vi "AprilTagFieldLayout_New2026Welded.vi"() -> (3 "AprilTagFieldLayout":T1={"AprilTagMap"={}, "FieldLength"=0.0, "FieldWidth"=0.0, "OriginPosition "=enum."kBlueAllianceWallRightSide,", "OriginPose3d"={"Translation3d"={"X"=0.0, "Y"=0.0, "Z"=0.0}, "Rotation3d"={"Q_quaternion"={"R"=1.0, "V"=[0.0, 0.0, 0.0]}}}} {"OriginPose3d"."Translation3d"."Z" format="%14.3f"; "OriginPose3d"."Translation3d"."Y" format="%14.3f"; "OriginPose3d"."Translation3d"."X" format="%14.3f"})   [LabVIEW 2019, in "Trajectory_Library.lvlib"]
doc: "Define the FRC 2026 April Tag field layout.\n\nInputs:\n <none>\n\nOutputs:\n -- AprilTagFieldLayout -- AprilTagFieldLayout -- Data cluster containing field definition."
uses:
  TypeDef/AprilTagFieldLayout.ctl
  TypeDef/AprilTag.ctl
  TypeDef/POSE3D.ctl
  TypeDef/TRANSLATION3D.ctl
  TypeDef/ROTATION3D.ctl
  TypeDef/QUATERNION.ctl
  Enum/AprilTagFieldLayoutOrignPosition_ENUM.ctl
  AprilTag_GetAll.vi
  Quaternion_Normalize.vi
  Quaternion_New_Default.vi
  Trajectory_Library.lvlib
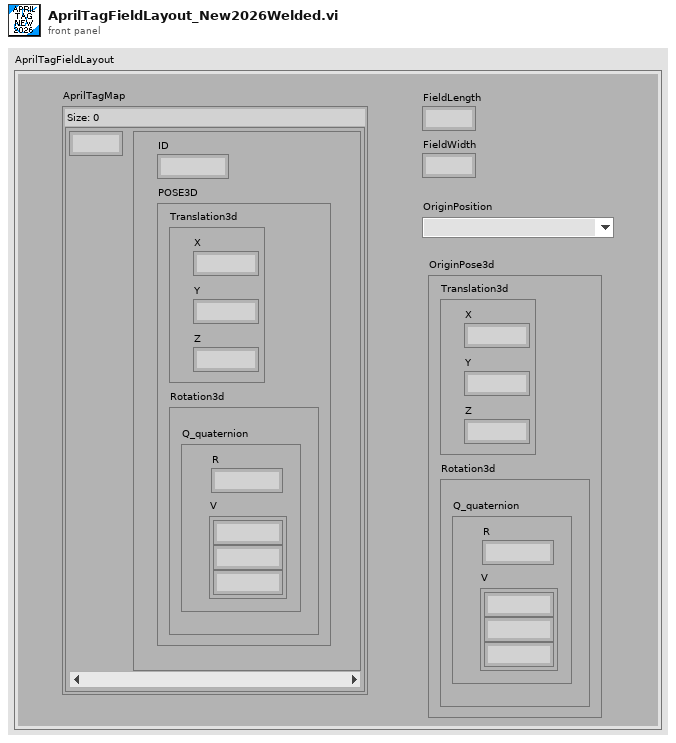
[diagram p1: front panel]
types:
  T1 = typedef "Trajectory_Library.lvlib/AprilTagFieldLayout.ctl" = cluster{"AprilTagMap":map{i32, T2}, "FieldLength":dbl, "FieldWidth":dbl, "OriginPosition ":T7, "OriginPose3d":T3}
  T2 = typedef "Trajectory_Library.lvlib/AprilTag.ctl" = cluster{"ID":i32, "POSE3D":T3}
  T3 = typedef "Trajectory_Library.lvlib/POSE3D.ctl" = cluster{"Translation3d":T4, "Rotation3d":T5}
  T4 = typedef "Trajectory_Library.lvlib/TRANSLATION3D.ctl" = cluster{"X":dbl, "Y":dbl, "Z":dbl}
  T5 = typedef "Trajectory_Library.lvlib/ROTATION3D.ctl" = cluster{"Q_quaternion":T6}
  T6 = typedef "Trajectory_Library.lvlib/QUATERNION.ctl" = cluster{"R":dbl, "V":dbl[]}
  T7 = typedef "Trajectory_Library.lvlib/AprilTagFieldLayoutOrignPosition_ENUM.ctl" = enum16{"kBlueAllianceWallRightSide,", "kRedAllianceWallRightSide,"}
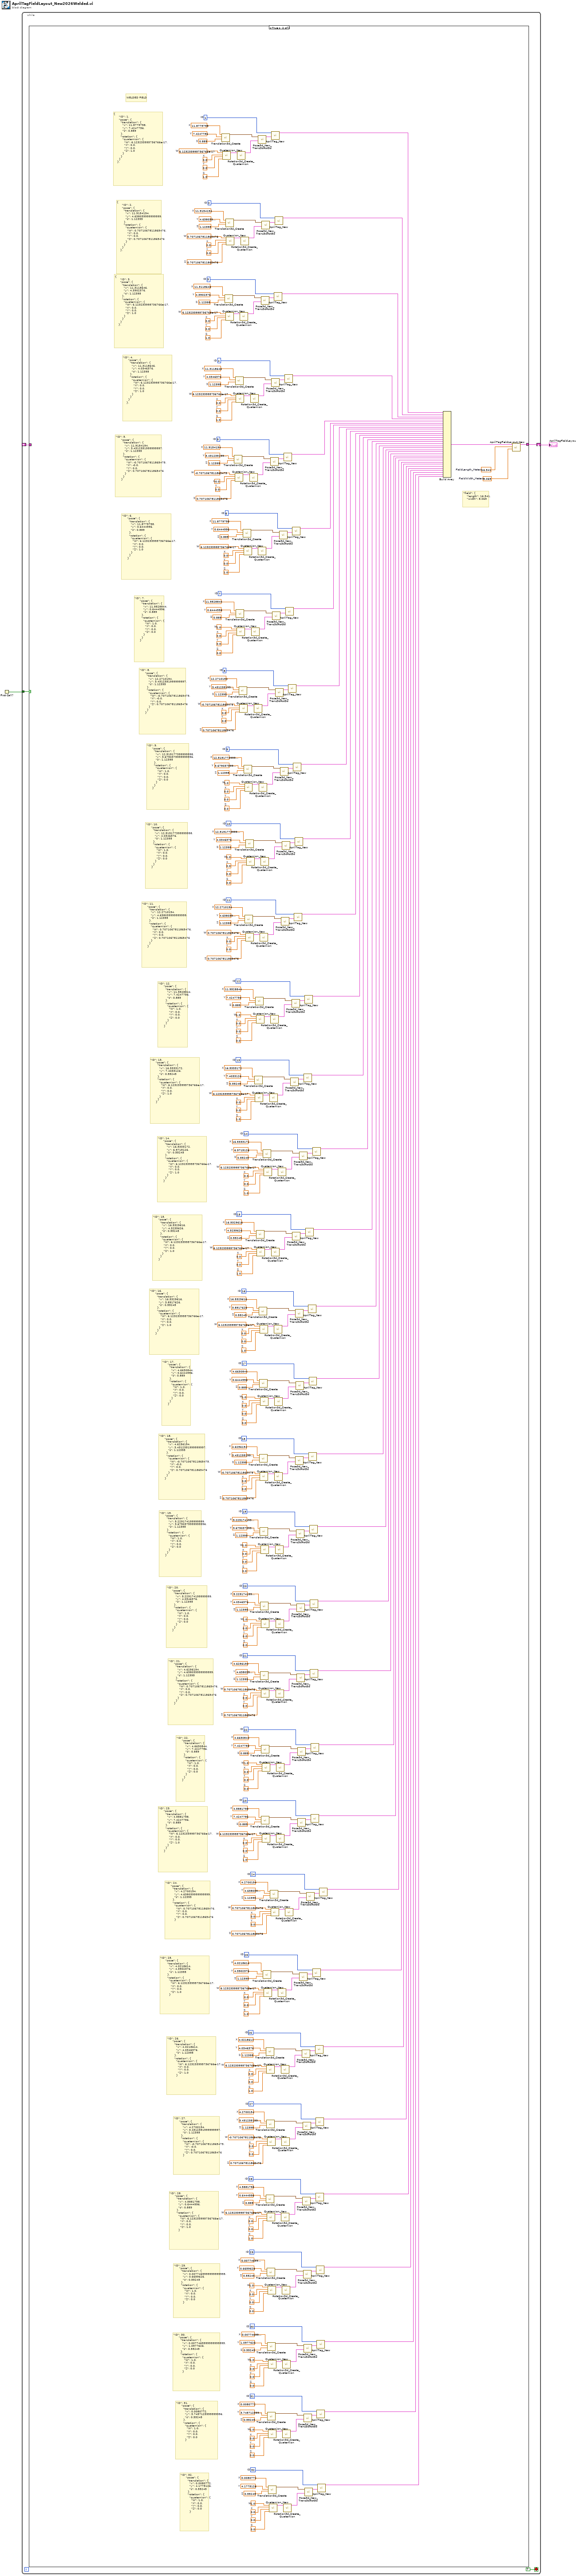
[diagram p0: block diagram]
diagram:
  n1 = First Call?() -> (First Call?: T/F=w1:bool)
  n2 = while {
    shift-right: [w6] -> w2
    shift-left: _ -> [w3]
    tunnel: w1 -> [w4]
    stop <- TRUE stop-if-true
    n3 = case shown="True" w4 {
      tunnel: [w7 w427] -> w6
      tunnel: w3 -> [w7 _]
      frame False {
      }
      frame True {
        w19 = 32  # ID
        w21 = 0.0080772  # X
        w22 = 4.1775126  # Y
        w23 = 0.55245  # Z
        w20 = 1.0  # W
        w24 = 0.0  # X
        w25 = 0.0  # Y
        w26 = 0.0  # Z
        w31 = 31  # ID
        w33 = 0.0080772  # X
        w34 = 3.7457125999999996  # Y
        w35 = 0.55245  # Z
        w32 = 1.0  # W
        w36 = 0.0  # X
        w37 = 0.0  # Y
        w38 = 0.0  # Z
        w43 = 30  # ID
        w45 = 0.0077469999999999995  # X
        w46 = 1.0977626  # Y
        w47 = 0.55245  # Z
        w44 = 1.0  # W
        w48 = 0.0  # X
        w49 = 0.0  # Y
        w50 = 0.0  # Z
        w55 = 29  # ID
        w57 = 0.0077469999999999995  # X
        w58 = 0.6659626  # Y
        w59 = 0.55245  # Z
        w56 = 1.0  # W
        w60 = 0.0  # X
        w61 = 0.0  # Y
        w62 = 0.0  # Z
        w67 = 28  # ID
        w69 = 4.5881798  # X
        w70 = 0.6444996  # Y
        w71 = 0.889  # Z
        w68 = 6.123233995736766e-17  # W
        w72 = 0.0  # X
        w73 = 0.0  # Y
        w74 = 1.0  # Z
        w79 = 27  # ID
        w81 = 4.2700194  # X
        w82 = 3.4312351999999997  # Y
        w83 = 1.12395  # Z
        w80 = -0.7071067811865475  # W
        w84 = 0.0  # X
        w85 = 0.0  # Y
        w86 = 0.7071067811865476  # Z
        w91 = 26  # ID
        w93 = 4.0218614  # X
        w94 = 4.0346376  # Y
        w95 = 1.12395  # Z
        w92 = 6.123233995736766e-17  # W
        w96 = 0.0  # X
        w97 = 0.0  # Y
        w98 = 1.0  # Z
        w103 = 25  # ID
        w105 = 4.0218614  # X
        w106 = 4.3902376  # Y
        w107 = 1.12395  # Z
        w104 = 6.123233995736766e-17  # W
        w108 = 0.0  # X
        w109 = 0.0  # Y
        w110 = 1.0  # Z
        w115 = 24  # ID
        w117 = 4.2700194  # X
        w118 = 4.638039999999999  # Y
        w119 = 1.12395  # Z
        w116 = 0.7071067811865476  # W
        w120 = 0.0  # X
        w121 = 0.0  # Y
        w122 = 0.7071067811865476  # Z
        w127 = 23  # ID
        w129 = 4.5881798  # X
        w130 = 7.4247756  # Y
        w131 = 0.889  # Z
        w128 = 6.123233995736766e-17  # W
        w132 = 0.0  # X
        w133 = 0.0  # Y
        w134 = 1.0  # Z
        w145 = 22  # ID
        w147 = 4.6630844  # X
        w148 = 7.4247756  # Y
        w149 = 0.889  # Z
        w146 = 1.0  # W
        w150 = 0.0  # X
        w151 = 0.0  # Y
        w152 = 0.0  # Z
        w157 = 21  # ID
        w159 = 4.6256194  # X
        w160 = 4.638039999999999  # Y
        w161 = 1.12395  # Z
        w158 = 0.7071067811865476  # W
        w162 = 0.0  # X
        w163 = 0.0  # Y
        w164 = 0.7071067811865476  # Z
        w169 = 20  # ID
        w171 = 5.229174199999999  # X
        w172 = 4.0346376  # Y
        w173 = 1.12395  # Z
        w170 = 1.0  # W
        w174 = 0.0  # X
        w175 = 0.0  # Y
        w176 = 0.0  # Z
        w181 = 19  # ID
        w183 = 5.229174199999999  # X
        w184 = 3.6790375999999996  # Y
        w185 = 1.12395  # Z
        w182 = 1.0  # W
        w186 = 0.0  # X
        w187 = 0.0  # Y
        w188 = 0.0  # Z
        w193 = 18  # ID
        w195 = 4.6256194  # X
        w196 = 3.4312351999999997  # Y
        w197 = 1.12395  # Z
        w194 = -0.7071067811865475  # W
        w198 = 0.0  # X
        w199 = 0.0  # Y
        w200 = 0.7071067811865476  # Z
        w205 = 17  # ID
        w207 = 4.6630844  # X
        w208 = 0.6444996  # Y
        w209 = 0.889  # Z
        w206 = 1.0  # W
        w210 = 0.0  # X
        w211 = 0.0  # Y
        w212 = 0.0  # Z
        w225 = 16  # ID
        w227 = 16.5329616  # X
        w228 = 3.8917626  # Y
        w229 = 0.55245  # Z
        w226 = 6.123233995736766e-17  # W
        w230 = 0.0  # X
        w231 = 0.0  # Y
        w232 = 1.0  # Z
        w237 = 15  # ID
        w239 = 16.5329616  # X
        w240 = 4.3235626  # Y
        w241 = 0.55245  # Z
        w238 = 6.123233995736766e-17  # W
        w242 = 0.0  # X
        w243 = 0.0  # Y
        w244 = 1.0  # Z
        w249 = 14  # ID
        w251 = 16.5333172  # X
        w252 = 6.9715126  # Y
        w253 = 0.55245  # Z
        w250 = 6.123233995736766e-17  # W
        w254 = 0.0  # X
        w255 = 0.0  # Y
        w256 = 1.0  # Z
        w261 = 13  # ID
        w263 = 16.5333172  # X
        w264 = 7.4033126  # Y
        w265 = 0.55245  # Z
        w262 = 6.123233995736766e-17  # W
        w266 = 0.0  # X
        w267 = 0.0  # Y
        w268 = 1.0  # Z
        w273 = 12  # ID
        w275 = 11.9528844  # X
        w276 = 7.4247756  # Y
        w277 = 0.889  # Z
        w274 = 1.0  # W
        w278 = 0.0  # X
        w279 = 0.0  # Y
        w280 = 0.0  # Z
        w285 = 11  # ID
        w287 = 12.2710194  # X
        w288 = 4.638039999999999  # Y
        w289 = 1.12395  # Z
        w286 = 0.7071067811865476  # W
        w290 = 0.0  # X
        w291 = 0.0  # Y
        w292 = 0.7071067811865476  # Z
        w297 = 10  # ID
        w299 = 12.519177399999998  # X
        w300 = 4.0346376  # Y
        w301 = 1.12395  # Z
        w298 = 1.0  # W
        w302 = 0.0  # X
        w303 = 0.0  # Y
        w304 = 0.0  # Z
        w309 = 9  # ID
        w311 = 12.519177399999998  # X
        w312 = 3.6790375999999996  # Y
        w313 = 1.12395  # Z
        w310 = 1.0  # W
        w314 = 0.0  # X
        w315 = 0.0  # Y
        w316 = 0.0  # Z
        w330 = 8  # ID
        w332 = 12.2710194  # X
        w333 = 3.4312351999999997  # Y
        w334 = 1.12395  # Z
        w331 = -0.7071067811865475  # W
        w335 = 0.0  # X
        w336 = 0.0  # Y
        w337 = 0.7071067811865476  # Z
        w342 = 7  # ID
        w344 = 11.9528844  # X
        w345 = 0.6444996  # Y
        w346 = 0.889  # Z
        w343 = 1.0  # W
        w347 = 0.0  # X
        w348 = 0.0  # Y
        w349 = 0.0  # Z
        w354 = 6  # ID
        w356 = 11.8779798  # X
        w357 = 0.6444996  # Y
        w358 = 0.889  # Z
        w355 = 6.123233995736766e-17  # W
        w359 = 0.0  # X
        w360 = 0.0  # Y
        w361 = 1.0  # Z
        w366 = 5  # ID
        w368 = 11.9154194  # X
        w369 = 3.4312351999999997  # Y
        w370 = 1.12395  # Z
        w367 = -0.7071067811865475  # W
        w371 = -0.0  # X
        w372 = 0.0  # Y
        w373 = 0.7071067811865476  # Z
        w378 = 4  # ID
        w380 = 11.3118646  # X
        w381 = 4.0346376  # Y
        w382 = 1.12395  # Z
        w379 = 6.123233995736766e-17  # W
        w383 = 0.0  # X
        w384 = 0.0  # Y
        w385 = 1.0  # Z
        w390 = 3  # ID
        w392 = 11.3118646  # X
        w393 = 4.3902376  # Y
        w394 = 1.12395  # Z
        w391 = 6.123233995736766e-17  # W
        w395 = 0.0  # X
        w396 = 0.0  # Y
        w397 = 1.0  # Z
        w402 = 2  # ID
        w404 = 11.9154194  # X
        w405 = 4.638039999999999  # Y
        w406 = 1.12395  # Z
        w403 = 0.7071067811865476  # W
        w407 = 0.0  # X
        w408 = 0.0  # Y
        w409 = 0.7071067811865476  # Z
        w414 = 1  # ID
        w416 = 11.8779798  # X
        w417 = 7.4247756  # Y
        w418 = 0.889  # Z
        w415 = 6.123233995736766e-17  # W
        w419 = 0.0  # X
        w420 = 0.0  # Y
        w421 = 1.0  # Z
        w425 = 8.069  # FieldWidth_Meters
        w426 = 16.541  # FieldLength_Meters
        # "\"field\": {\n    \"length\": 16.541,\n    \"width\": 8.069"
        # "\"ID\": 32,\n      \"pose\": {\n        \"translation\": {\n          \"x\": 0.0080772,\n          \"y\": 4.1775126,\n          \"z\": 0.55245\n        },\n        \"rotation\": {\n          \"quaternion\": {\n            \"W\": 1.0,\n            \"X\": 0.0,\n            \"Y\": 0.0,\n            \"Z\": 0.0\n          }"
        # "\"ID\": 31,\n      \"pose\": {\n        \"translation\": {\n          \"x\": 0.0080772,\n          \"y\": 3.7457125999999996,\n          \"z\": 0.55245\n        },\n        \"rotation\": {\n          \"quaternion\": {\n            \"W\": 1.0,\n            \"X\": 0.0,\n            \"Y\": 0.0,\n            \"Z\": 0.0\n          }"
        # "\"ID\": 30,\n      \"pose\": {\n        \"translation\": {\n          \"x\": 0.0077469999999999995,\n          \"y\": 1.0977626,\n          \"z\": 0.55245\n        },\n        \"rotation\": {\n          \"quaternion\": {\n            \"W\": 1.0,\n            \"X\": 0.0,\n            \"Y\": 0.0,\n            \"Z\": 0.0\n          }"
        # "\"ID\": 29,\n      \"pose\": {\n        \"translation\": {\n          \"x\": 0.0077469999999999995,\n          \"y\": 0.6659626,\n          \"z\": 0.55245\n        },\n        \"rotation\": {\n          \"quaternion\": {\n            \"W\": 1.0,\n            \"X\": 0.0,\n            \"Y\": 0.0,\n            \"Z\": 0.0\n          }"
        # "\"ID\": 28,\n      \"pose\": {\n        \"translation\": {\n          \"x\": 4.5881798,\n          \"y\": 0.6444996,\n          \"z\": 0.889\n        },\n        \"rotation\": {\n          \"quaternion\": {\n            \"W\": 6.123233995736766e-17,\n            \"X\": 0.0,\n            \"Y\": 0.0,\n            \"Z\": 1.0\n          }"
        # "\"ID\": 27,\n      \"pose\": {\n        \"translation\": {\n          \"x\": 4.2700194,\n          \"y\": 3.4312351999999997,\n          \"z\": 1.12395\n        },\n        \"rotation\": {\n          \"quaternion\": {\n            \"W\": -0.7071067811865475,\n            \"X\": -0.0,\n            \"Y\": 0.0,\n            \"Z\": 0.7071067811865476\n          }"
        # "\"ID\": 26,\n      \"pose\": {\n        \"translation\": {\n          \"x\": 4.0218614,\n          \"y\": 4.0346376,\n          \"z\": 1.12395\n        },\n        \"rotation\": {\n          \"quaternion\": {\n            \"W\": 6.123233995736766e-17,\n            \"X\": 0.0,\n            \"Y\": 0.0,\n            \"Z\": 1.0\n          }"
        # "\"ID\": 25,\n      \"pose\": {\n        \"translation\": {\n          \"x\": 4.0218614,\n          \"y\": 4.3902376,\n          \"z\": 1.12395\n        },\n        \"rotation\": {\n          \"quaternion\": {\n            \"W\": 6.123233995736766e-17,\n            \"X\": 0.0,\n            \"Y\": 0.0,\n            \"Z\": 1.0\n          }"
        # "\"ID\": 24,\n      \"pose\": {\n        \"translation\": {\n          \"x\": 4.2700194,\n          \"y\": 4.638039999999999,\n          \"z\": 1.12395\n        },\n        \"rotation\": {\n          \"quaternion\": {\n            \"W\": 0.7071067811865476,\n            \"X\": 0.0,\n            \"Y\": 0.0,\n            \"Z\": 0.7071067811865476\n          }"
        # "\"ID\": 23,\n      \"pose\": {\n        \"translation\": {\n          \"x\": 4.5881798,\n          \"y\": 7.4247756,\n          \"z\": 0.889\n        },\n        \"rotation\": {\n          \"quaternion\": {\n            \"W\": 6.123233995736766e-17,\n            \"X\": 0.0,\n            \"Y\": 0.0,\n            \"Z\": 1.0\n          }\n        }\n      }"
        # "\"ID\": 22,\n      \"pose\": {\n        \"translation\": {\n          \"x\": 4.6630844,\n          \"y\": 7.4247756,\n          \"z\": 0.889\n        },\n        \"rotation\": {\n          \"quaternion\": {\n            \"W\": 1.0,\n            \"X\": 0.0,\n            \"Y\": 0.0,\n            \"Z\": 0.0\n          }\n        }\n      }"
        # "\"ID\": 21,\n      \"pose\": {\n        \"translation\": {\n          \"x\": 4.6256194,\n          \"y\": 4.638039999999999,\n          \"z\": 1.12395\n        },\n        \"rotation\": {\n          \"quaternion\": {\n            \"W\": 0.7071067811865476,\n            \"X\": 0.0,\n            \"Y\": 0.0,\n            \"Z\": 0.7071067811865476\n          }\n        }\n      }"
        # "\"ID\": 20,\n      \"pose\": {\n        \"translation\": {\n          \"x\": 5.229174199999999,\n          \"y\": 4.0346376,\n          \"z\": 1.12395\n        },\n        \"rotation\": {\n          \"quaternion\": {\n            \"W\": 1.0,\n            \"X\": 0.0,\n            \"Y\": 0.0,\n            \"Z\": 0.0\n          }\n        }\n      }"
        # "\"ID\": 19,\n      \"pose\": {\n        \"translation\": {\n          \"x\": 5.229174199999999,\n          \"y\": 3.6790375999999996,\n          \"z\": 1.12395\n        },\n        \"rotation\": {\n          \"quaternion\": {\n            \"W\": 1.0,\n            \"X\": 0.0,\n            \"Y\": 0.0,\n            \"Z\": 0.0\n          }\n        }\n      }"
        # "\"ID\": 18,\n      \"pose\": {\n        \"translation\": {\n          \"x\": 4.6256194,\n          \"y\": 3.4312351999999997,\n          \"z\": 1.12395\n        },\n        \"rotation\": {\n          \"quaternion\": {\n            \"W\": -0.7071067811865475,\n            \"X\": -0.0,\n            \"Y\": 0.0,\n            \"Z\": 0.7071067811865476\n          }\n        }\n      }"
        # "\"ID\": 17,\n      \"pose\": {\n        \"translation\": {\n          \"x\": 4.6630844,\n          \"y\": 0.6444996,\n          \"z\": 0.889\n        },\n        \"rotation\": {\n          \"quaternion\": {\n            \"W\": 1.0,\n            \"X\": 0.0,\n            \"Y\": 0.0,\n            \"Z\": 0.0\n          }\n        }\n      }"
        # "\"ID\": 16,\n      \"pose\": {\n        \"translation\": {\n          \"x\": 16.5329616,\n          \"y\": 3.8917626,\n          \"z\": 0.55245\n        },\n        \"rotation\": {\n          \"quaternion\": {\n            \"W\": 6.123233995736766e-17,\n            \"X\": 0.0,\n            \"Y\": 0.0,\n            \"Z\": 1.0\n          }\n        }\n      }"
        # "\"ID\": 15,\n      \"pose\": {\n        \"translation\": {\n          \"x\": 16.5329616,\n          \"y\": 4.3235626,\n          \"z\": 0.55245\n        },\n        \"rotation\": {\n          \"quaternion\": {\n            \"W\": 6.123233995736766e-17,\n            \"X\": 0.0,\n            \"Y\": 0.0,\n            \"Z\": 1.0\n          }\n        }\n      }"
        # "\"ID\": 14,\n      \"pose\": {\n        \"translation\": {\n          \"x\": 16.5333172,\n          \"y\": 6.9715126,\n          \"z\": 0.55245\n        },\n        \"rotation\": {\n          \"quaternion\": {\n            \"W\": 6.123233995736766e-17,\n            \"X\": 0.0,\n            \"Y\": 0.0,\n            \"Z\": 1.0\n          }\n        }\n      }"
        # "\"ID\": 13,\n      \"pose\": {\n        \"translation\": {\n          \"x\": 16.5333172,\n          \"y\": 7.4033126,\n          \"z\": 0.55245\n        },\n        \"rotation\": {\n          \"quaternion\": {\n            \"W\": 6.123233995736766e-17,\n            \"X\": 0.0,\n            \"Y\": 0.0,\n            \"Z\": 1.0\n          }\n        }\n      }"
        # "\"ID\": 12,\n      \"pose\": {\n        \"translation\": {\n          \"x\": 11.9528844,\n          \"y\": 7.4247756,\n          \"z\": 0.889\n        },\n        \"rotation\": {\n          \"quaternion\": {\n            \"W\": 1.0,\n            \"X\": 0.0,\n            \"Y\": 0.0,\n            \"Z\": 0.0\n          }\n        }\n      }"
        # "\"ID\": 11,\n      \"pose\": {\n        \"translation\": {\n          \"x\": 12.2710194,\n          \"y\": 4.638039999999999,\n          \"z\": 1.12395\n        },\n        \"rotation\": {\n          \"quaternion\": {\n            \"W\": 0.7071067811865476,\n            \"X\": 0.0,\n            \"Y\": 0.0,\n            \"Z\": 0.7071067811865476\n          }\n        }\n      }"
        # "\"ID\": 10,\n      \"pose\": {\n        \"translation\": {\n          \"x\": 12.519177399999998,\n          \"y\": 4.0346376,\n          \"z\": 1.12395\n        },\n        \"rotation\": {\n          \"quaternion\": {\n            \"W\": 1.0,\n            \"X\": 0.0,\n            \"Y\": 0.0,\n            \"Z\": 0.0\n          }\n        }\n      }"
        # "\"ID\": 9,\n      \"pose\": {\n        \"translation\": {\n          \"x\": 12.519177399999998,\n          \"y\": 3.6790375999999996,\n          \"z\": 1.12395\n        },\n        \"rotation\": {\n          \"quaternion\": {\n            \"W\": 1.0,\n            \"X\": 0.0,\n            \"Y\": 0.0,\n            \"Z\": 0.0\n          }\n        }\n      }"
        # "\"ID\": 8,\n      \"pose\": {\n        \"translation\": {\n          \"x\": 12.2710194,\n          \"y\": 3.4312351999999997,\n          \"z\": 1.12395\n        },\n        \"rotation\": {\n          \"quaternion\": {\n            \"W\": -0.7071067811865475,\n            \"X\": -0.0,\n            \"Y\": 0.0,\n            \"Z\": 0.7071067811865476\n          }\n        }\n      }"
        # "\"ID\": 7,\n      \"pose\": {\n        \"translation\": {\n          \"x\": 11.9528844,\n          \"y\": 0.6444996,\n          \"z\": 0.889\n        },\n        \"rotation\": {\n          \"quaternion\": {\n            \"W\": 1.0,\n            \"X\": 0.0,\n            \"Y\": 0.0,\n            \"Z\": 0.0\n          }\n        }\n      }"
        # "\"ID\": 6,\n      \"pose\": {\n        \"translation\": {\n          \"x\": 11.8779798,\n          \"y\": 0.6444996,\n          \"z\": 0.889\n        },\n        \"rotation\": {\n          \"quaternion\": {\n            \"W\": 6.123233995736766e-17,\n            \"X\": 0.0,\n            \"Y\": 0.0,\n            \"Z\": 1.0\n          }\n        }\n      }"
        # "\"ID\": 5,\n      \"pose\": {\n        \"translation\": {\n          \"x\": 11.9154194,\n          \"y\": 3.4312351999999997,\n          \"z\": 1.12395\n        },\n        \"rotation\": {\n          \"quaternion\": {\n            \"W\": -0.7071067811865475,\n            \"X\": -0.0,\n            \"Y\": 0.0,\n            \"Z\": 0.7071067811865476\n          }\n        }\n      }"
        # "\"ID\": 4,\n      \"pose\": {\n        \"translation\": {\n          \"x\": 11.3118646,\n          \"y\": 4.0346376,\n          \"z\": 1.12395\n        },\n        \"rotation\": {\n          \"quaternion\": {\n            \"W\": 6.123233995736766e-17,\n            \"X\": 0.0,\n            \"Y\": 0.0,\n            \"Z\": 1.0\n          }\n        }\n      }\n    },"
        # "{\n      \"ID\": 3,\n      \"pose\": {\n        \"translation\": {\n          \"x\": 11.3118646,\n          \"y\": 4.3902376,\n          \"z\": 1.12395\n        },\n        \"rotation\": {\n          \"quaternion\": {\n            \"W\": 6.123233995736766e-17,\n            \"X\": 0.0,\n            \"Y\": 0.0,\n            \"Z\": 1.0\n          }\n        }\n      }\n    },"
        # "{\n      \"ID\": 2,\n      \"pose\": {\n        \"translation\": {\n          \"x\": 11.9154194,\n          \"y\": 4.638039999999999,\n          \"z\": 1.12395\n        },\n        \"rotation\": {\n          \"quaternion\": {\n            \"W\": 0.7071067811865476,\n            \"X\": 0.0,\n            \"Y\": 0.0,\n            \"Z\": 0.7071067811865476\n          }\n        }\n      }\n    },"
        # "{\n      \"ID\": 1,\n      \"pose\": {\n        \"translation\": {\n          \"x\": 11.8779798,\n          \"y\": 7.4247756,\n          \"z\": 0.889\n        },\n        \"rotation\": {\n          \"quaternion\": {\n            \"W\": 6.123233995736766e-17,\n            \"X\": 0.0,\n            \"Y\": 0.0,\n            \"Z\": 1.0\n          }\n        }\n      }\n    },"
        # "WELDED FIELD"
        n4 = call "Translation3d_Create.vi"("Z"=w418, "Y"=w417, "X"=w416) -> ("TRANSLATION3D"=w424:T4)  [unwired: 8 in]
        n5 = call "Quaternion_New.vi"("Z"=w421, "Y"=w420, "X"=w419, "W"=w415) -> ("out Quaternion"=w422:T6)  [unwired: 7 in]
        n6 = call "Translation3d_Create.vi"("Z"=w394, "Y"=w393, "X"=w392) -> ("TRANSLATION3D"=w400:T4)  [unwired: 8 in]
        n7 = call "Translation3d_Create.vi"("Z"=w406, "Y"=w405, "X"=w404) -> ("TRANSLATION3D"=w412:T4)  [unwired: 8 in]
        n8 = call "Quaternion_New.vi"("Z"=w397, "Y"=w396, "X"=w395, "W"=w391) -> ("out Quaternion"=w398:T6)  [unwired: 7 in]
        n9 = call "Quaternion_New.vi"("Z"=w409, "Y"=w408, "X"=w407, "W"=w403) -> ("out Quaternion"=w410:T6)  [unwired: 7 in]
        n10 = call "Translation3d_Create.vi"("Z"=w370, "Y"=w369, "X"=w368) -> ("TRANSLATION3D"=w376:T4)  [unwired: 8 in]
        n11 = call "Quaternion_New.vi"("Z"=w373, "Y"=w372, "X"=w371, "W"=w367) -> ("out Quaternion"=w374:T6)  [unwired: 7 in]
        n12 = call "Translation3d_Create.vi"("Z"=w382, "Y"=w381, "X"=w380) -> ("TRANSLATION3D"=w388:T4)  [unwired: 8 in]
        n13 = call "Quaternion_New.vi"("Z"=w385, "Y"=w384, "X"=w383, "W"=w379) -> ("out Quaternion"=w386:T6)  [unwired: 7 in]
        n14 = call "Translation3d_Create.vi"("Z"=w346, "Y"=w345, "X"=w344) -> ("TRANSLATION3D"=w352:T4)  [unwired: 8 in]
        n15 = call "Quaternion_New.vi"("Z"=w349, "Y"=w348, "X"=w347, "W"=w343) -> ("out Quaternion"=w350:T6)  [unwired: 7 in]
        n16 = call "Rotation3d_Create_Quaternion.vi"("Quaternion"=w422) -> ("Rotation3d"=w423:T5)  [unwired: 10 in]
        n17 = call "Translation3d_Create.vi"("Z"=w334, "Y"=w333, "X"=w332) -> ("TRANSLATION3D"=w340:T4)  [unwired: 8 in]
        n18 = call "Quaternion_New.vi"("Z"=w337, "Y"=w336, "X"=w335, "W"=w331) -> ("out Quaternion"=w338:T6)  [unwired: 7 in]
        n19 = call "Rotation3d_Create_Quaternion.vi"("Quaternion"=w398) -> ("Rotation3d"=w399:T5)  [unwired: 10 in]
        n20 = call "Rotation3d_Create_Quaternion.vi"("Quaternion"=w410) -> ("Rotation3d"=w411:T5)  [unwired: 10 in]
        n21 = call "Translation3d_Create.vi"("Z"=w358, "Y"=w357, "X"=w356) -> ("TRANSLATION3D"=w364:T4)  [unwired: 8 in]
        n22 = call "Quaternion_New.vi"("Z"=w361, "Y"=w360, "X"=w359, "W"=w355) -> ("out Quaternion"=w362:T6)  [unwired: 7 in]
        n23 = call "Translation3d_Create.vi"("Z"=w313, "Y"=w312, "X"=w311) -> ("TRANSLATION3D"=w319:T4)  [unwired: 8 in]
        n24 = call "Quaternion_New.vi"("Z"=w316, "Y"=w315, "X"=w314, "W"=w310) -> ("out Quaternion"=w317:T6)  [unwired: 7 in]
        n25 = call "Translation3d_Create.vi"("Z"=w289, "Y"=w288, "X"=w287) -> ("TRANSLATION3D"=w295:T4)  [unwired: 8 in]
        n26 = call "Translation3d_Create.vi"("Z"=w301, "Y"=w300, "X"=w299) -> ("TRANSLATION3D"=w307:T4)  [unwired: 8 in]
        n27 = call "Quaternion_New.vi"("Z"=w292, "Y"=w291, "X"=w290, "W"=w286) -> ("out Quaternion"=w293:T6)  [unwired: 7 in]
        n28 = call "Quaternion_New.vi"("Z"=w304, "Y"=w303, "X"=w302, "W"=w298) -> ("out Quaternion"=w305:T6)  [unwired: 7 in]
        n29 = call "Rotation3d_Create_Quaternion.vi"("Quaternion"=w374) -> ("Rotation3d"=w375:T5)  [unwired: 10 in]
        n30 = call "Rotation3d_Create_Quaternion.vi"("Quaternion"=w386) -> ("Rotation3d"=w387:T5)  [unwired: 10 in]
        n31 = call "Rotation3d_Create_Quaternion.vi"("Quaternion"=w350) -> ("Rotation3d"=w351:T5)  [unwired: 10 in]
        n32 = call "Rotation3d_Create_Quaternion.vi"("Quaternion"=w338) -> ("Rotation3d"=w339:T5)  [unwired: 10 in]
        n33 = call "Translation3d_Create.vi"("Z"=w265, "Y"=w264, "X"=w263) -> ("TRANSLATION3D"=w271:T4)  [unwired: 8 in]
        n34 = call "Quaternion_New.vi"("Z"=w268, "Y"=w267, "X"=w266, "W"=w262) -> ("out Quaternion"=w269:T6)  [unwired: 7 in]
        n35 = call "Translation3d_Create.vi"("Z"=w277, "Y"=w276, "X"=w275) -> ("TRANSLATION3D"=w283:T4)  [unwired: 8 in]
        n36 = call "Quaternion_New.vi"("Z"=w280, "Y"=w279, "X"=w278, "W"=w274) -> ("out Quaternion"=w281:T6)  [unwired: 7 in]
        n37 = call "Translation3d_Create.vi"("Z"=w241, "Y"=w240, "X"=w239) -> ("TRANSLATION3D"=w247:T4)  [unwired: 8 in]
        n38 = call "Quaternion_New.vi"("Z"=w244, "Y"=w243, "X"=w242, "W"=w238) -> ("out Quaternion"=w245:T6)  [unwired: 7 in]
        n39 = call "Pose3d_New_Trans3dRot3d.vi"("Rotation3d"=w423, "Translation3d"=w424) -> ("outPose3d"=w413:T3)  [unwired: 9 in]
        n40 = call "Rotation3d_Create_Quaternion.vi"("Quaternion"=w362) -> ("Rotation3d"=w363:T5)  [unwired: 10 in]
        n41 = call "Rotation3d_Create_Quaternion.vi"("Quaternion"=w317) -> ("Rotation3d"=w318:T5)  [unwired: 10 in]
        n42 = call "Translation3d_Create.vi"("Z"=w229, "Y"=w228, "X"=w227) -> ("TRANSLATION3D"=w235:T4)  [unwired: 8 in]
        n43 = call "Translation3d_Create.vi"("Z"=w197, "Y"=w196, "X"=w195) -> ("TRANSLATION3D"=w203:T4)  [unwired: 8 in]
        n44 = call "Translation3d_Create.vi"("Z"=w209, "Y"=w208, "X"=w207) -> ("TRANSLATION3D"=w215:T4)  [unwired: 8 in]
        n45 = call "Quaternion_New.vi"("Z"=w232, "Y"=w231, "X"=w230, "W"=w226) -> ("out Quaternion"=w233:T6)  [unwired: 7 in]
        n46 = call "Rotation3d_Create_Quaternion.vi"("Quaternion"=w293) -> ("Rotation3d"=w294:T5)  [unwired: 10 in]
        n47 = call "Quaternion_New.vi"("Z"=w200, "Y"=w199, "X"=w198, "W"=w194) -> ("out Quaternion"=w201:T6)  [unwired: 7 in]
        n48 = call "Translation3d_Create.vi"("Z"=w185, "Y"=w184, "X"=w183) -> ("TRANSLATION3D"=w191:T4)  [unwired: 8 in]
        n49 = call "Quaternion_New.vi"("Z"=w212, "Y"=w211, "X"=w210, "W"=w206) -> ("out Quaternion"=w213:T6)  [unwired: 7 in]
        n50 = call "Translation3d_Create.vi"("Z"=w173, "Y"=w172, "X"=w171) -> ("TRANSLATION3D"=w179:T4)  [unwired: 8 in]
        n51 = call "Translation3d_Create.vi"("Z"=w161, "Y"=w160, "X"=w159) -> ("TRANSLATION3D"=w167:T4)  [unwired: 8 in]
        n52 = call "Rotation3d_Create_Quaternion.vi"("Quaternion"=w305) -> ("Rotation3d"=w306:T5)  [unwired: 10 in]
        n53 = call "Quaternion_New.vi"("Z"=w188, "Y"=w187, "X"=w186, "W"=w182) -> ("out Quaternion"=w189:T6)  [unwired: 7 in]
        n54 = call "Pose3d_New_Trans3dRot3d.vi"("Rotation3d"=w399, "Translation3d"=w400) -> ("outPose3d"=w389:T3)  [unwired: 9 in]
        n55 = call "Quaternion_New.vi"("Z"=w176, "Y"=w175, "X"=w174, "W"=w170) -> ("out Quaternion"=w177:T6)  [unwired: 7 in]
        n56 = call "Quaternion_New.vi"("Z"=w164, "Y"=w163, "X"=w162, "W"=w158) -> ("out Quaternion"=w165:T6)  [unwired: 7 in]
        n57 = call "Translation3d_Create.vi"("Z"=w149, "Y"=w148, "X"=w147) -> ("TRANSLATION3D"=w155:T4)  [unwired: 8 in]
        n58 = call "Translation3d_Create.vi"("Z"=w131, "Y"=w130, "X"=w129) -> ("TRANSLATION3D"=w137:T4)  [unwired: 8 in]
        n59 = call "Pose3d_New_Trans3dRot3d.vi"("Rotation3d"=w411, "Translation3d"=w412) -> ("outPose3d"=w401:T3)  [unwired: 9 in]
        n60 = call "Quaternion_New.vi"("Z"=w152, "Y"=w151, "X"=w150, "W"=w146) -> ("out Quaternion"=w153:T6)  [unwired: 7 in]
        n61 = call "Quaternion_New.vi"("Z"=w134, "Y"=w133, "X"=w132, "W"=w128) -> ("out Quaternion"=w135:T6)  [unwired: 7 in]
        n62 = call "Translation3d_Create.vi"("Z"=w253, "Y"=w252, "X"=w251) -> ("TRANSLATION3D"=w259:T4)  [unwired: 8 in]
        n63 = call "Translation3d_Create.vi"("Z"=w107, "Y"=w106, "X"=w105) -> ("TRANSLATION3D"=w113:T4)  [unwired: 8 in]
        n64 = call "Quaternion_New.vi"("Z"=w256, "Y"=w255, "X"=w254, "W"=w250) -> ("out Quaternion"=w257:T6)  [unwired: 7 in]
        n65 = call "Quaternion_New.vi"("Z"=w110, "Y"=w109, "X"=w108, "W"=w104) -> ("out Quaternion"=w111:T6)  [unwired: 7 in]
        n66 = call "Translation3d_Create.vi"("Z"=w95, "Y"=w94, "X"=w93) -> ("TRANSLATION3D"=w101:T4)  [unwired: 8 in]
        n67 = call "Translation3d_Create.vi"("Z"=w71, "Y"=w70, "X"=w69) -> ("TRANSLATION3D"=w77:T4)  [unwired: 8 in]
        n68 = call "Translation3d_Create.vi"("Z"=w83, "Y"=w82, "X"=w81) -> ("TRANSLATION3D"=w89:T4)  [unwired: 8 in]
        n69 = call "Quaternion_New.vi"("Z"=w98, "Y"=w97, "X"=w96, "W"=w92) -> ("out Quaternion"=w99:T6)  [unwired: 7 in]
        n70 = call "Quaternion_New.vi"("Z"=w74, "Y"=w73, "X"=w72, "W"=w68) -> ("out Quaternion"=w75:T6)  [unwired: 7 in]
        n71 = call "Translation3d_Create.vi"("Z"=w59, "Y"=w58, "X"=w57) -> ("TRANSLATION3D"=w65:T4)  [unwired: 8 in]
        n72 = call "Quaternion_New.vi"("Z"=w86, "Y"=w85, "X"=w84, "W"=w80) -> ("out Quaternion"=w87:T6)  [unwired: 7 in]
        n73 = call "Translation3d_Create.vi"("Z"=w47, "Y"=w46, "X"=w45) -> ("TRANSLATION3D"=w53:T4)  [unwired: 8 in]
        n74 = call "Translation3d_Create.vi"("Z"=w35, "Y"=w34, "X"=w33) -> ("TRANSLATION3D"=w41:T4)  [unwired: 8 in]
        n75 = call "Quaternion_New.vi"("Z"=w62, "Y"=w61, "X"=w60, "W"=w56) -> ("out Quaternion"=w63:T6)  [unwired: 7 in]
        n76 = call "Quaternion_New.vi"("Z"=w50, "Y"=w49, "X"=w48, "W"=w44) -> ("out Quaternion"=w51:T6)  [unwired: 7 in]
        n77 = call "Quaternion_New.vi"("Z"=w38, "Y"=w37, "X"=w36, "W"=w32) -> ("out Quaternion"=w39:T6)  [unwired: 7 in]
        n78 = call "Translation3d_Create.vi"("Z"=w23, "Y"=w22, "X"=w21) -> ("TRANSLATION3D"=w29:T4)  [unwired: 8 in]
        n79 = call "Quaternion_New.vi"("Z"=w26, "Y"=w25, "X"=w24, "W"=w20) -> ("out Quaternion"=w27:T6)  [unwired: 7 in]
        n80 = call "Rotation3d_Create_Quaternion.vi"("Quaternion"=w269) -> ("Rotation3d"=w270:T5)  [unwired: 10 in]
        n81 = call "Translation3d_Create.vi"("Z"=w119, "Y"=w118, "X"=w117) -> ("TRANSLATION3D"=w125:T4)  [unwired: 8 in]
        n82 = call "Pose3d_New_Trans3dRot3d.vi"("Rotation3d"=w375, "Translation3d"=w376) -> ("outPose3d"=w365:T3)  [unwired: 9 in]
        n83 = call "Rotation3d_Create_Quaternion.vi"("Quaternion"=w281) -> ("Rotation3d"=w282:T5)  [unwired: 10 in]
        n84 = call "Quaternion_New.vi"("Z"=w122, "Y"=w121, "X"=w120, "W"=w116) -> ("out Quaternion"=w123:T6)  [unwired: 7 in]
        n85 = call "AprilTag_New.vi"("POSE3D"=w413, "ID"=w414) -> ("AprilTag"=w327:T2)  [unwired: 9 in]
        n86 = call "Rotation3d_Create_Quaternion.vi"("Quaternion"=w245) -> ("Rotation3d"=w246:T5)  [unwired: 10 in]
        n87 = call "Pose3d_New_Trans3dRot3d.vi"("Rotation3d"=w387, "Translation3d"=w388) -> ("outPose3d"=w377:T3)  [unwired: 9 in]
        n88 = call "Pose3d_New_Trans3dRot3d.vi"("Rotation3d"=w351, "Translation3d"=w352) -> ("outPose3d"=w341:T3)  [unwired: 9 in]
        n89 = call "AprilTag_New.vi"("POSE3D"=w389, "ID"=w390) -> ("AprilTag"=w325:T2)  [unwired: 9 in]
        n90 = call "Rotation3d_Create_Quaternion.vi"("Quaternion"=w233) -> ("Rotation3d"=w234:T5)  [unwired: 10 in]
        n91 = call "Rotation3d_Create_Quaternion.vi"("Quaternion"=w201) -> ("Rotation3d"=w202:T5)  [unwired: 10 in]
        n92 = call "Rotation3d_Create_Quaternion.vi"("Quaternion"=w213) -> ("Rotation3d"=w214:T5)  [unwired: 10 in]
        n93 = call "AprilTag_New.vi"("POSE3D"=w401, "ID"=w402) -> ("AprilTag"=w326:T2)  [unwired: 9 in]
        n94 = call "Pose3d_New_Trans3dRot3d.vi"("Rotation3d"=w339, "Translation3d"=w340) -> ("outPose3d"=w329:T3)  [unwired: 9 in]
        n95 = call "Rotation3d_Create_Quaternion.vi"("Quaternion"=w189) -> ("Rotation3d"=w190:T5)  [unwired: 10 in]
        n96 = call "Rotation3d_Create_Quaternion.vi"("Quaternion"=w177) -> ("Rotation3d"=w178:T5)  [unwired: 10 in]
        n97 = call "Rotation3d_Create_Quaternion.vi"("Quaternion"=w165) -> ("Rotation3d"=w166:T5)  [unwired: 10 in]
        n98 = call "Rotation3d_Create_Quaternion.vi"("Quaternion"=w153) -> ("Rotation3d"=w154:T5)  [unwired: 10 in]
        n99 = call "Rotation3d_Create_Quaternion.vi"("Quaternion"=w135) -> ("Rotation3d"=w136:T5)  [unwired: 10 in]
        n100 = call "Rotation3d_Create_Quaternion.vi"("Quaternion"=w257) -> ("Rotation3d"=w258:T5)  [unwired: 10 in]
        n101 = call "Rotation3d_Create_Quaternion.vi"("Quaternion"=w111) -> ("Rotation3d"=w112:T5)  [unwired: 10 in]
        n102 = call "Pose3d_New_Trans3dRot3d.vi"("Rotation3d"=w363, "Translation3d"=w364) -> ("outPose3d"=w353:T3)  [unwired: 9 in]
        n103 = call "Pose3d_New_Trans3dRot3d.vi"("Rotation3d"=w318, "Translation3d"=w319) -> ("outPose3d"=w308:T3)  [unwired: 9 in]
        n104 = call "Pose3d_New_Trans3dRot3d.vi"("Rotation3d"=w294, "Translation3d"=w295) -> ("outPose3d"=w284:T3)  [unwired: 9 in]
        n105 = call "Rotation3d_Create_Quaternion.vi"("Quaternion"=w99) -> ("Rotation3d"=w100:T5)  [unwired: 10 in]
        n106 = call "Rotation3d_Create_Quaternion.vi"("Quaternion"=w75) -> ("Rotation3d"=w76:T5)  [unwired: 10 in]
        n107 = call "Rotation3d_Create_Quaternion.vi"("Quaternion"=w87) -> ("Rotation3d"=w88:T5)  [unwired: 10 in]
        n108 = call "Pose3d_New_Trans3dRot3d.vi"("Rotation3d"=w306, "Translation3d"=w307) -> ("outPose3d"=w296:T3)  [unwired: 9 in]
        n109 = call "Rotation3d_Create_Quaternion.vi"("Quaternion"=w63) -> ("Rotation3d"=w64:T5)  [unwired: 10 in]
        n110 = call "Rotation3d_Create_Quaternion.vi"("Quaternion"=w51) -> ("Rotation3d"=w52:T5)  [unwired: 10 in]
        n111 = call "Rotation3d_Create_Quaternion.vi"("Quaternion"=w39) -> ("Rotation3d"=w40:T5)  [unwired: 10 in]
        n112 = call "Rotation3d_Create_Quaternion.vi"("Quaternion"=w27) -> ("Rotation3d"=w28:T5)  [unwired: 10 in]
        n113 = call "AprilTag_New.vi"("POSE3D"=w365, "ID"=w366) -> ("AprilTag"=w323:T2)  [unwired: 9 in]
        n114 = call "AprilTag_New.vi"("POSE3D"=w377, "ID"=w378) -> ("AprilTag"=w324:T2)  [unwired: 9 in]
        n115 = call "Rotation3d_Create_Quaternion.vi"("Quaternion"=w123) -> ("Rotation3d"=w124:T5)  [unwired: 10 in]
        n116 = call "AprilTag_New.vi"("POSE3D"=w341, "ID"=w342) -> ("AprilTag"=w321:T2)  [unwired: 9 in]
        n117 = call "AprilTag_New.vi"("POSE3D"=w329, "ID"=w330) -> ("AprilTag"=w320:T2)  [unwired: 9 in]
        n118 = call "Pose3d_New_Trans3dRot3d.vi"("Rotation3d"=w270, "Translation3d"=w271) -> ("outPose3d"=w260:T3)  [unwired: 9 in]
        n119 = call "Pose3d_New_Trans3dRot3d.vi"("Rotation3d"=w282, "Translation3d"=w283) -> ("outPose3d"=w272:T3)  [unwired: 9 in]
        n120 = call "AprilTag_New.vi"("POSE3D"=w353, "ID"=w354) -> ("AprilTag"=w322:T2)  [unwired: 9 in]
        n121 = call "Pose3d_New_Trans3dRot3d.vi"("Rotation3d"=w246, "Translation3d"=w247) -> ("outPose3d"=w236:T3)  [unwired: 9 in]
        n122 = call "AprilTag_New.vi"("POSE3D"=w308, "ID"=w309) -> ("AprilTag"=w223:T2)  [unwired: 9 in]
        n123 = call "AprilTag_New.vi"("POSE3D"=w284, "ID"=w285) -> ("AprilTag"=w221:T2)  [unwired: 9 in]
        n124 = call "AprilTag_New.vi"("POSE3D"=w296, "ID"=w297) -> ("AprilTag"=w222:T2)  [unwired: 9 in]
        n125 = call "Pose3d_New_Trans3dRot3d.vi"("Rotation3d"=w234, "Translation3d"=w235) -> ("outPose3d"=w224:T3)  [unwired: 9 in]
        n126 = call "Pose3d_New_Trans3dRot3d.vi"("Rotation3d"=w202, "Translation3d"=w203) -> ("outPose3d"=w192:T3)  [unwired: 9 in]
        n127 = call "Pose3d_New_Trans3dRot3d.vi"("Rotation3d"=w214, "Translation3d"=w215) -> ("outPose3d"=w204:T3)  [unwired: 9 in]
        n128 = call "Pose3d_New_Trans3dRot3d.vi"("Rotation3d"=w190, "Translation3d"=w191) -> ("outPose3d"=w180:T3)  [unwired: 9 in]
        n129 = call "Pose3d_New_Trans3dRot3d.vi"("Rotation3d"=w178, "Translation3d"=w179) -> ("outPose3d"=w168:T3)  [unwired: 9 in]
        n130 = call "Pose3d_New_Trans3dRot3d.vi"("Rotation3d"=w166, "Translation3d"=w167) -> ("outPose3d"=w156:T3)  [unwired: 9 in]
        n131 = call "Pose3d_New_Trans3dRot3d.vi"("Rotation3d"=w154, "Translation3d"=w155) -> ("outPose3d"=w144:T3)  [unwired: 9 in]
        n132 = call "Pose3d_New_Trans3dRot3d.vi"("Rotation3d"=w136, "Translation3d"=w137) -> ("outPose3d"=w126:T3)  [unwired: 9 in]
        n133 = call "Pose3d_New_Trans3dRot3d.vi"("Rotation3d"=w258, "Translation3d"=w259) -> ("outPose3d"=w248:T3)  [unwired: 9 in]
        n134 = call "Pose3d_New_Trans3dRot3d.vi"("Rotation3d"=w112, "Translation3d"=w113) -> ("outPose3d"=w102:T3)  [unwired: 9 in]
        n135 = call "Pose3d_New_Trans3dRot3d.vi"("Rotation3d"=w100, "Translation3d"=w101) -> ("outPose3d"=w90:T3)  [unwired: 9 in]
        n136 = call "Pose3d_New_Trans3dRot3d.vi"("Rotation3d"=w76, "Translation3d"=w77) -> ("outPose3d"=w66:T3)  [unwired: 9 in]
        n137 = call "Pose3d_New_Trans3dRot3d.vi"("Rotation3d"=w88, "Translation3d"=w89) -> ("outPose3d"=w78:T3)  [unwired: 9 in]
        n138 = call "Pose3d_New_Trans3dRot3d.vi"("Rotation3d"=w64, "Translation3d"=w65) -> ("outPose3d"=w54:T3)  [unwired: 9 in]
        n139 = call "AprilTag_New.vi"("POSE3D"=w260, "ID"=w261) -> ("AprilTag"=w219:T2)  [unwired: 9 in]
        n140 = call "Pose3d_New_Trans3dRot3d.vi"("Rotation3d"=w52, "Translation3d"=w53) -> ("outPose3d"=w42:T3)  [unwired: 9 in]
        n141 = call "Pose3d_New_Trans3dRot3d.vi"("Rotation3d"=w40, "Translation3d"=w41) -> ("outPose3d"=w30:T3)  [unwired: 9 in]
        n142 = call "Pose3d_New_Trans3dRot3d.vi"("Rotation3d"=w28, "Translation3d"=w29) -> ("outPose3d"=w18:T3)  [unwired: 9 in]
        n143 = call "AprilTag_New.vi"("POSE3D"=w272, "ID"=w273) -> ("AprilTag"=w220:T2)  [unwired: 9 in]
        n144 = call "AprilTag_New.vi"("POSE3D"=w236, "ID"=w237) -> ("AprilTag"=w217:T2)  [unwired: 9 in]
        n145 = call "Pose3d_New_Trans3dRot3d.vi"("Rotation3d"=w124, "Translation3d"=w125) -> ("outPose3d"=w114:T3)  [unwired: 9 in]
        n146 = call "AprilTag_New.vi"("POSE3D"=w224, "ID"=w225) -> ("AprilTag"=w216:T2)  [unwired: 9 in]
        n147 = call "AprilTag_New.vi"("POSE3D"=w192, "ID"=w193) -> ("AprilTag"=w142:T2)  [unwired: 9 in]
        n148 = call "AprilTag_New.vi"("POSE3D"=w204, "ID"=w205) -> ("AprilTag"=w143:T2)  [unwired: 9 in]
        n149 = call "AprilTag_New.vi"("POSE3D"=w180, "ID"=w181) -> ("AprilTag"=w141:T2)  [unwired: 9 in]
        n150 = call "AprilTag_New.vi"("POSE3D"=w168, "ID"=w169) -> ("AprilTag"=w140:T2)  [unwired: 9 in]
        n151 = call "AprilTag_New.vi"("POSE3D"=w156, "ID"=w157) -> ("AprilTag"=w139:T2)  [unwired: 9 in]
        n152 = call "AprilTag_New.vi"("POSE3D"=w144, "ID"=w145) -> ("AprilTag"=w138:T2)  [unwired: 9 in]
        n153 = call "AprilTag_New.vi"("POSE3D"=w126, "ID"=w127) -> ("AprilTag"=w17:T2)  [unwired: 9 in]
        n154 = call "AprilTag_New.vi"("POSE3D"=w248, "ID"=w249) -> ("AprilTag"=w218:T2)  [unwired: 9 in]
        n155 = call "AprilTag_New.vi"("POSE3D"=w102, "ID"=w103) -> ("AprilTag"=w15:T2)  [unwired: 9 in]
        n156 = call "AprilTag_New.vi"("POSE3D"=w90, "ID"=w91) -> ("AprilTag"=w14:T2)  [unwired: 9 in]
        n157 = call "AprilTag_New.vi"("POSE3D"=w66, "ID"=w67) -> ("AprilTag"=w12:T2)  [unwired: 9 in]
        n158 = call "AprilTag_New.vi"("POSE3D"=w78, "ID"=w79) -> ("AprilTag"=w13:T2)  [unwired: 9 in]
        n159 = call "AprilTag_New.vi"("POSE3D"=w54, "ID"=w55) -> ("AprilTag"=w11:T2)  [unwired: 9 in]
        n160 = call "AprilTag_New.vi"("POSE3D"=w42, "ID"=w43) -> ("AprilTag"=w10:T2)  [unwired: 9 in]
        n161 = call "AprilTag_New.vi"("POSE3D"=w30, "ID"=w31) -> ("AprilTag"=w9:T2)  [unwired: 9 in]
        n162 = call "AprilTag_New.vi"("POSE3D"=w18, "ID"=w19) -> ("AprilTag"=w8:T2)  [unwired: 9 in]
        n163 = call "AprilTag_New.vi"("POSE3D"=w114, "ID"=w115) -> ("AprilTag"=w16:T2)  [unwired: 9 in]
        n164 = Build Array(w327, w326, w325, w324, w323, w322, w321, w320, w223, w222, w221, w220, w219, w218, w217, w216, w143, w142, w141, w140, w139, w138, w17, w16, w15, w14, w13, w12, w11, w10, w9, w8) -> (w328:T2[])
        n165 = call "AprilTagFieldLayout_New.vi"("FieldWidth_Meters"=w425, "FieldLength_Meters"=w426, "AprilTags"=w328) -> ("AprilTagFieldLayout"=w427:T1)  [unwired: 8 in]
      }
    }
  }
  "AprilTagFieldLayout" <- w2
